vi "Get Variables.vi"(8 "error in (no error)":errorcluster, 11 "For Loop in":refnum<class "Structure Loop.lvclass">) -> (0 "error out":errorcluster, 2 "Variables":variant, 3 "For Loop out":refnum<class "Structure Loop.lvclass">)   [LabVIEW 2019, in "Structure Loop.lvclass"]
uses:
  Structure Loop.lvclass
  Structure Loop.lvclass/Structure Loop.ctl
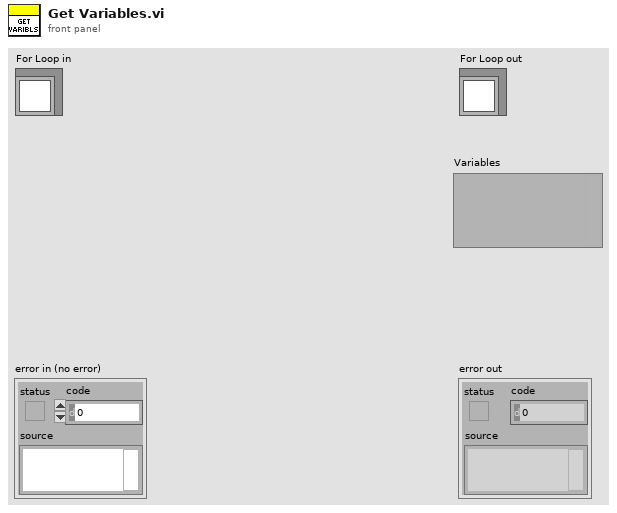
[diagram p1: front panel]
types:
  T1 = typedef "Structure Loop.lvclass/Variables.ctl" = cluster{"Continue?":bool, "element":string, "elements":variant}
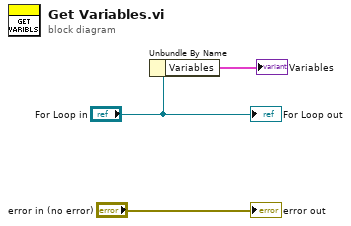
[diagram p0: block diagram]
diagram:
  n1 = Unbundle By Name("For Loop in") -> ("Variables"=→"Variables":T1)
  "error out" <- "error in (no error)"
  "For Loop out" <- "For Loop in"
